vi "SiosIfmGetMeasurementSettings.vi"(0 "devNumber":i32) -> (1 "success":i32, 2 "MeasurementSettings":T1={"SendChannel1Data"=FALSE, "SendChannel2Data"=FALSE, "SendChannel3Data"=FALSE, "SendChannel4Data"=FALSE, "SendLengthValues"=FALSE, "SendSinCosData"=FALSE, "SendCircleData"=FALSE, "SendTestPattern"=FALSE, "SendClockCounterValue"=FALSE, "SendSampleCounterValue"=FALSE, "FilterSettings"=enum."Filter off", "OutputWordRate"=0})   [LabVIEW 2009]
uses:
  siosifm.dll
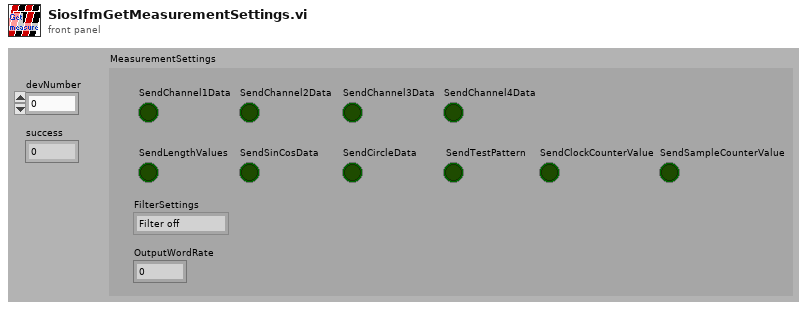
[diagram p1: front panel]
types:
  T1 = cluster{"SendChannel1Data":bool, "SendChannel2Data":bool, "SendChannel3Data":bool, "SendChannel4Data":bool, "SendLengthValues":bool, "SendSinCosData":bool, "SendCircleData":bool, "SendTestPattern":bool, "SendClockCounterValue":bool, "SendSampleCounterValue":bool, "FilterSettings":enum32{"Auto filter", "Filter off", "Filter user specified"}, "OutputWordRate":i32}
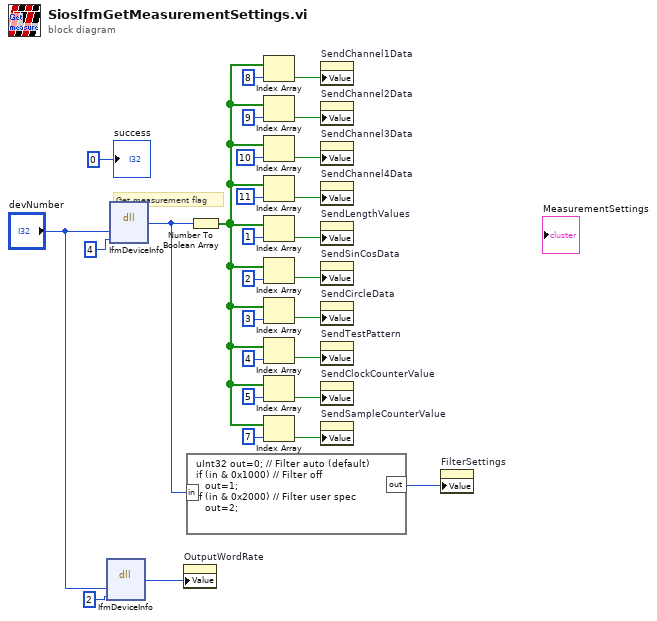
[diagram p0: block diagram]
diagram:
  # "Get measurement flag"
  n1 = dll-call lib="D:/Support/Labview/RE-10/SIOS_IfmDLL/siosifm.dll" fn="IfmDeviceInfo"("devNumber"="devNumber", "requestedInfoFlag"=u32 2) -> (w10:i32)  [unwired: 5 in, 2 out]
  n2 = dll-call lib="D:/Support/Labview/RE-10/SIOS_IfmDLL/siosifm.dll" fn="IfmDeviceInfo"("devNumber"="devNumber", "requestedInfoFlag"=u32 4) -> (w4:u32)  [unwired: 5 in, 2 out]
  n3 = property on="OutputWordRate" class="DigitalWert (strikt)"("Value"=w10) -> ()  [unwired: 2 in, 2 out]
  n4 = formula code="uInt32 out=0; // Filter auto (default)\nif (in & 0x1000) // Filter off\n   out=1;\nif (in & 0x2000) // Filter user spec\n   out=2;"("in"=w4) -> ("out"=w3:u32)
  n5 = Number To Boolean Array(number=w4) -> (Boolean array=w5:bool[])
  n6 = Index Array(array=w5, index=8 ("Index")) -> (element=w28:bool)
  n7 = Index Array(array=w5, index=9 ("Index")) -> (element=w27:bool)
  n8 = Index Array(array=w5, index=10 ("Index")) -> (element=w26:bool)
  n9 = Index Array(array=w5, index=11 ("Index")) -> (element=w25:bool)
  n10 = Index Array(array=w5, index=1 ("Index")) -> (element=w24:bool)
  n11 = Index Array(array=w5, index=2 ("Index")) -> (element=w14:bool)
  n12 = Index Array(array=w5, index=3 ("Index")) -> (element=w13:bool)
  n13 = Index Array(array=w5, index=4 ("Index")) -> (element=w12:bool)
  n14 = Index Array(array=w5, index=5 ("Index")) -> (element=w7:bool)
  n15 = Index Array(array=w5, index=7 ("Index")) -> (element=w6:bool)
  n16 = property on="SendChannel1Data" class="Boolesch (strikt)"("Value"=w28) -> ()  [unwired: 2 in, 2 out]
  n17 = property on="SendChannel2Data" class="Boolesch (strikt)"("Value"=w27) -> ()  [unwired: 2 in, 2 out]
  n18 = property on="SendChannel3Data" class="Boolesch (strikt)"("Value"=w26) -> ()  [unwired: 2 in, 2 out]
  n19 = property on="SendChannel4Data" class="Boolesch (strikt)"("Value"=w25) -> ()  [unwired: 2 in, 2 out]
  n20 = property on="SendLengthValues" class="Boolesch (strikt)"("Value"=w24) -> ()  [unwired: 2 in, 2 out]
  n21 = property on="SendSinCosData" class="Boolesch (strikt)"("Value"=w14) -> ()  [unwired: 2 in, 2 out]
  n22 = property on="SendCircleData" class="Boolesch (strikt)"("Value"=w13) -> ()  [unwired: 2 in, 2 out]
  n23 = property on="SendTestPattern" class="Boolesch (strikt)"("Value"=w12) -> ()  [unwired: 2 in, 2 out]
  n24 = property on="SendClockCounterValue" class="Boolesch (strikt)"("Value"=w7) -> ()  [unwired: 2 in, 2 out]
  n25 = property on="SendSampleCounterValue" class="Boolesch (strikt)"("Value"=w6) -> ()  [unwired: 2 in, 2 out]
  n26 = property on="FilterSettings" class="Enum (strikt)"("Value"=w3) -> ()  [unwired: 2 in, 2 out]
  "success" <- 0
